vi "Read Memory Location.vi"(8 "error in (no error)":errorcluster, 11 "VISA resource name":refnum<visa-resource-name>) -> (0 "error out":errorcluster, 2 "Memory Location":i32, 3 "VISA resource name out":refnum<visa-resource-name>)   [LabVIEW 2018, in "EFD Ultimus V.lvlib"]
doc: "Reads the current memory location that the dispenser is set to. \n\nHost Format: UA---\n\nReturn Format: D0ccc\nccc: The 3 digit memory location from 0-399."
uses:
  EFD Ultimus V.lvlib
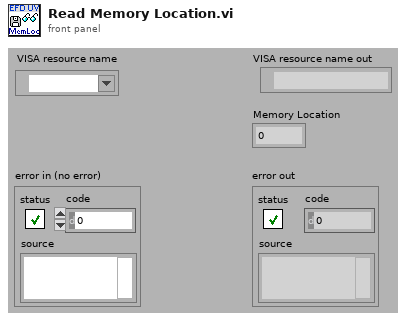
[diagram p1: front panel]
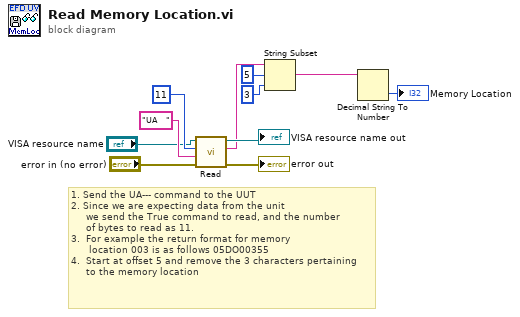
[diagram p0: block diagram]
diagram:
  # "1. Send the UA--- command to the UUT\n2. Since we are expecting data from the unit\n     we send the True command to read, and the number\n     of bytes to read as 11.\n3.  For example the return format for memory\n      location 003 is as follows 05DO00355\n4.  Start at offset 5 and remove the 3 characters pertaining\n     to the memory location"
  n1 = call "Read.vi"("error in (no error)"="error in (no error)", "Command To Write"="UA   ", "Bytes to Read (11)"=u32 11 ("bytes to read"), "VISA resource name"="VISA resource name") -> ("error out"=→"error out":errorcluster, "Ultimus V Feedback Data"=w5:string, "VISA resource name out"=→"VISA resource name out":refnum<visa-resource-name>)  [unwired: 5 out]
  n2 = String Subset(string=w5, offset (0)=5, length (rest)=3 ("length (rest)")) -> (substring=w4:string)
  n3 = Decimal String To Number(string=w4) -> (number=→"Memory Location":i32)  [unwired: 3 out]
